vi "Axis offsets.vi"(8 "error in":errorcluster, 10 "Axis offsets increment":dbl[](array[numeric])=[0.0, 0.0, 0.0, 0.0, 0.0, 0.0]) -> (0 "error out":errorcluster, 2 "Axis offsets":dbl[](array[numeric]))   [LabVIEW 2013]
panel:
  # "Axis offsets specify a fixed offset applied to the stage axis positions.    This VI specifies a change in the axis offsets, which is more typically desired.  This results in a read/write of the shared variable, and the new value is returned as a result.  This is specifically to fine-tune the home position when additional information is available, such as from ASAP, and should not be used as a general way to offset the pose.  See \"Home position\".  In particular, this can be used to make the Rz axis intersect the Rx and Ry axes by adding additional X and Y offsets, and can be used to trim the home position of the stepper axes, especially Rx, which has no particular kinematic signification, since it is the last sequential link.  For the stepper axes, specifying an axis offset is similar to driving the axis to a position and then using the \"set zero\" button on the motion server, but axis offsets is currently exported over the net, and \"set zero\" isn't"
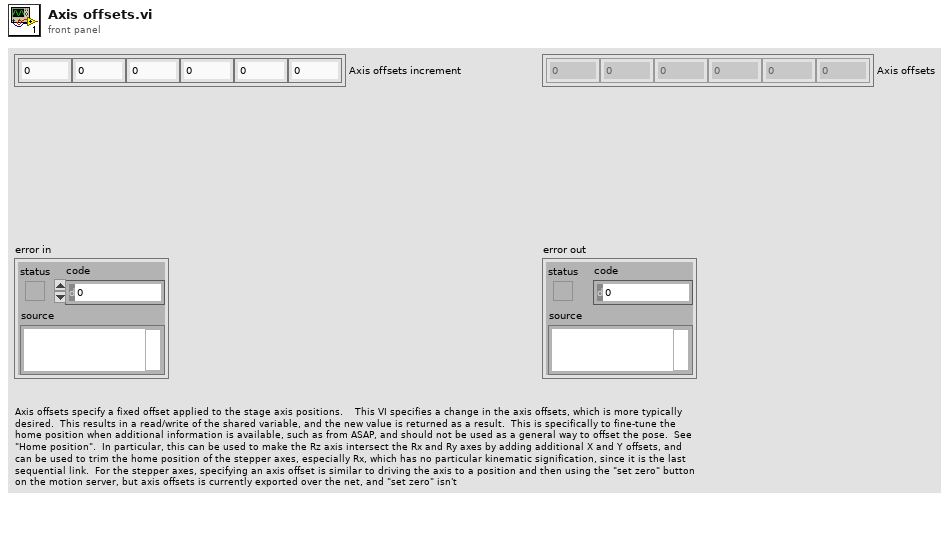
[diagram p1: front panel]
types:
  T1 = typedef "motion_variables.ctl" = cluster{"Motion command":refnum<k21>, "Motion status":refnum<k21>, "Emergency stop":refnum<k21>, "End transform":refnum<k21>, "Home position":refnum<k21>, "Axis offsets":refnum<k21>}
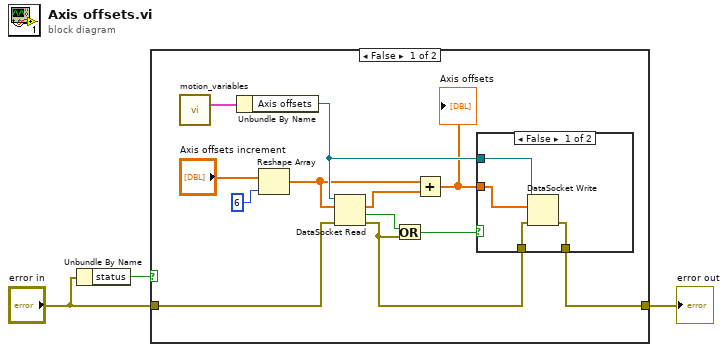
[diagram p0: block diagram]
diagram:
  n1 = Unbundle By Name("error in") -> ("status"=w1:bool)
  n2 = case shown="False" w1 {
    tunnel: [w14 w21] -> w3
    tunnel: "error in" -> [w12 w21]
    frame False {
      n3 = call "motion_variables.vi"() -> ("Motion variables"=w15:T1)  [unwired: 11 in]
      n4 = Unbundle By Name(w15) -> ("Axis offsets"=w13:refnum<k21>)
      n5 = Reshape Array("Axis offsets increment", 6 ("dimension size")) -> (w5:dbl[])
      n6 = DataSocket Read(8:w12, 10:w5, 11:w13) -> (0:w11:errorcluster, 1:w10:bool, 2:w8:dbl[])  [unwired: 2 in, 4 out]
      n7 = Or(x=w10, y=w11) -> (x .or. y?=w9:bool)
      n8 = Add(x=w5, y=w8) -> (x+y=w7:dbl[])
      "Axis offsets" <- w7
      n9 = case shown="False" w9 {
        tunnel: [w19 w20] -> w14
        tunnel: w7 -> [w16 _]
        tunnel: w13 -> [w18 _]
        tunnel: w11 -> [w17 w20]
        frame False {
          n10 = DataSocket Write(8:w17, 10:w16, 11:w18) -> (0:w19:errorcluster)  [unwired: 1 in, 2 out]
        }
        frame True {
        }
      }
    }
    frame True {
    }
  }
  "error out" <- w3
